vi "Exit.vi"(8 "error in (no error)":errorcluster, 11 "Old State":refnum<class "Localize.lvclass">) -> (0 "error out":errorcluster, 3 "New State":refnum<class "Localize.lvclass">)   [LabVIEW 2014, in "States.lvlib" / "Localize.lvclass"]
doc: "This is an abstract method. Override this method to define the behavior when you leave the state."
uses:
  Localize.lvclass
  <vilib>/ActorFramework/Message Enqueuer/Message Enqueuer.lvclass/Message Enqueuer.ctl
  <vilib>/ActorFramework/Message Enqueuer/Enqueue.vi
  <vilib>/ActorFramework/Message Priority Queue/Priority Enqueue.vi
  Process State/CoordinatorState.lvclass
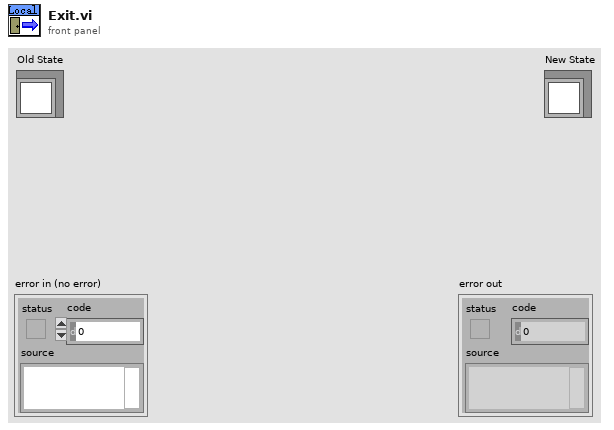
[diagram p1: front panel]
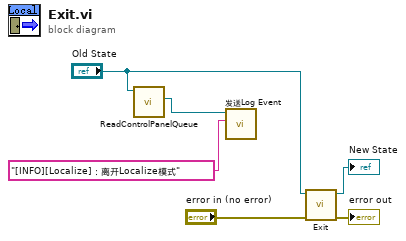
[diagram p0: block diagram]
diagram:
  n1 = call-dynamic "ReadControlPanelQueue.vi"("CoordinatorState输入"="Old State") -> ("操作者框架:消息待入队列"=w2:refnum<class "Message Enqueuer.lvclass">)  [unwired: 8 in, 2 out]
  n2 = call "发送Log Event.vi"("Event Text"="[INFO][Localize]：离开Localize模式", "消息待入队列"=w2) -> ()  [unwired: 8 in, 2 out]
  n3 = call-parent "Exit.vi"("error in (no error)"="error in (no error)", "Old State"="Old State") -> ("error out"=→"error out":errorcluster, "New State"=→"New State":refnum<class "Localize.lvclass">)  [unwired: 8 in]
